vi "FileInfo.vi"(0 "File/Folder Path":path, 11 "error in (no error)":errorcluster) -> (4 "ParentFolderPath":path, 6 "Type":string, 8 "Name":string, 10 "Size":string, 15 "error out":errorcluster)   [LabVIEW 2021, in "CustomSortPath.lvlib"]
doc: "This Vi gets the folder/file path as input and gives out the information like parent folder path,type,name and size."
uses:
  CustomSortPath.lvlib
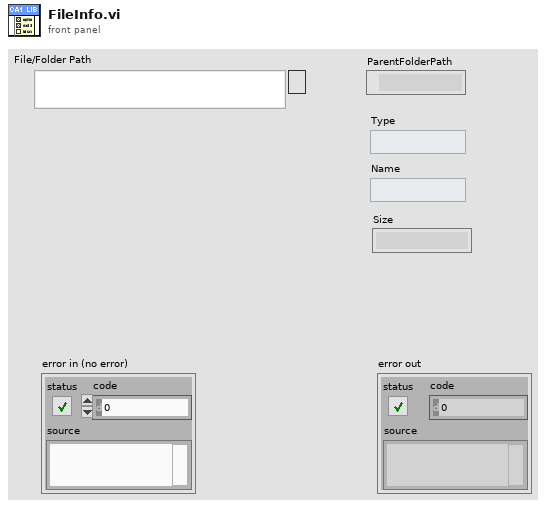
[diagram p1: front panel]
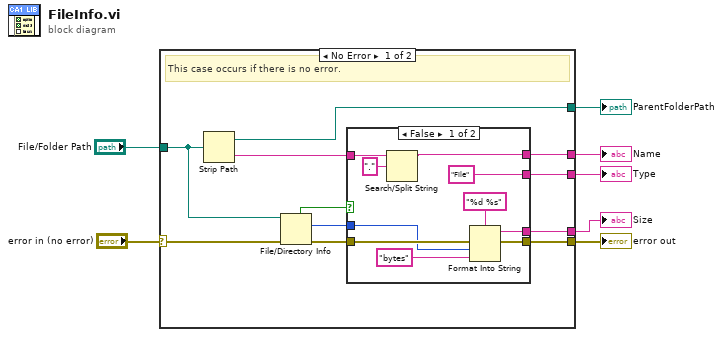
[diagram p0: block diagram]
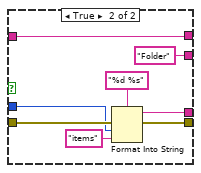
[diagram p2: hidden frame]
diagram:
  n1 = case shown="No Error" "error in (no error)" {
    selector: "error in (no error)" -> [w15 w37]
    tunnel: [w18 _] -> w7
    tunnel: [w17 _] -> w6
    tunnel: "File/Folder Path" -> [w16 _]
    tunnel: [w14 w37] -> w3
    tunnel: [w13 _] -> w2
    tunnel: [w12 _] -> w1
    frame No Error {
      # "This case occurs if there is no error."
      n2 = Strip Path(path=w16) -> (stripped path=w13:path, name=w11:string)
      n3 = File/Directory Info(path=w16, error in=w15) -> (directory=w9:bool, size=w8:i64, error out=w10:errorcluster)  [unwired: 4 out]
      n4 = case shown="False" w9 {
        tunnel: w11 -> [w28 w36]
        tunnel: [w26 w36] -> w18
        tunnel: ["File" ("substring before match") "Folder" ("substring before match")] -> w17
        tunnel: w10 -> [w25 w33]
        tunnel: [w22 w32] -> w14
        tunnel: [w20 w30] -> w12
        tunnel: w8 -> [w19 w29]
        frame False {
          n5 = Search/Split String(string=w28, search string/char (-)=".") -> (substring before match=w26:string)  [unwired: 1 in, 2 out]
          n6 = Format Into String(format string="%d %s", error in=w25, w19, "bytes" ("input 2")) -> (resulting string=w20:string, error out=w22:errorcluster)  [unwired: 1 in]
        }
        frame True {
          n7 = Format Into String(format string="%d %s", error in=w33, w29, "items" ("input 2")) -> (resulting string=w30:string, error out=w32:errorcluster)  [unwired: 1 in]
        }
      }
    }
    frame Error {
      # "This case occurs if there is any error."
    }
  }
  "Type" <- w6
  "Name" <- w7
  "error out" <- w3
  "ParentFolderPath" <- w2
  "Size" <- w1
